vi "Set VeriStand Error.vi"(6 "message":string, 8 "error in (no error)":errorcluster, 9 "key":string, 10 "errCode":i32(ring)=-307828 items=["Success"=0, "NoProjectOpen"=-307992, "SequenceCompileError"=-307988, "SessionAlreadyDeployed"=-307984, "SessionNotDeployed"=-307982, "SequenceNotFoundInSession"=-307981, "StimulusProfileSessionLocked"=-307980, "EmptyNodeName"=-307930, "NodeAlreadyExistsByName"=-307926, "NumberOfCoefficientsOutOfRange"=-307884, "DownloadFileError"=-307872, "IncorrectLogFileName"=-307871, "LogTriggerConditionSyntaxError"=-307868, "DuplicateLogSessionName"=-307867, "LogSessionNotFound"=-307865, "ChannelLengthMismatch"=-307830, "NodeNotFoundDuringCompile"=-307829, "ChannelNodeRemoved"=-307828, "NotAChannel"=-307825, "NotAWaveform"=-307824, "STIFileError"=-307784, "DependenciesCycle"=-307783, "ChannelNotFoundInLogFile"=-307782, "ChannelGroupNotFoundInLogFile"=-307781, "GatewayNotOnLocalhost"=-307780, "NotEnoughDynamicDataSharingSpace"=-307738, "TargetMissingDataSharingDevice"=-307737, "ChannelMappingsSizeMismatch"=-307728, "DuplicateChannelAliasMappings"=-307711, "NotAnInlineCustomDevice"=-307710, "IncompatibleModel"=-307703, "ModelDimensionMismatch"=-307702, "SLSCChassisLoadFailed"=-307691, "TargetDisabled"=-307689, "MismatchedLengths"=-307687, "TargetInvalid"=-307686, "ParameterNotFound"=-307685, "ServerPortAlreadyInUse"=-307684, "TargetDisconnected"=-307682, "ServiceConfigurationFile"=-307681, "ModelParameterFileParseError"=-307680, "NoActionRequired"=-307677, "InputParameterInvalid"=-307676, "HostRunningDifferentSystemDefinition"=-307671, "ChannelNotScalable"=-307668, "ChannelCannotBeFaulted"=-307666, "ChannelNotWritable"=-307665, "ChannelNotReadable"=-307664, "Timeout"=-307663, "NodeNotFound"=-307662, "SystemDefinitionDeploymentFailure"=-307661, "SystemDefinitionDeploymentTimeout"=-307660, "EmptyPassword"=-307659, "SystemDefinitionAlreadyActive"=-307658, "InvalidConfigurationPassword"=-307657, "NoSystemDefinitionLoaded"=-307656, "ComponentNotAvailable"=-307655, "NotDeployed"=-307654, "InvalidFile"=-307653, "FailedServerConnection"=-307652, "FunctionNotSupported"=-307651, "UnexpectedError"=-307650, "UnmappedAlias"=-307617, "InvalidStreamConditionForDataType"=-307554, "WaveformDataTypeMismatch"=-307553, "InvalidDaqPluginFile"=-307526, "FileVersionUnsupported"=-307525], 11 "Custom Device Item Ref in":T1 format="%.0x") -> (0 "error out":errorcluster, 1 "VeriStand Error out":errorcluster, 3 "Custom Device Item Ref out":T1 format="%.0x")   [LabVIEW 2017, in "Routing and Faulting Scripting.lvlib"]
uses:
  Routing and Faulting Scripting.lvlib
  <vilib>/NI Veristand/Custom Device API/Custom Device Item Ref.ctl
  NationalInstruments.VeriStand.SystemStorage
  <vilib>/NI Veristand/Custom Device API/Custom Device API.lvlib
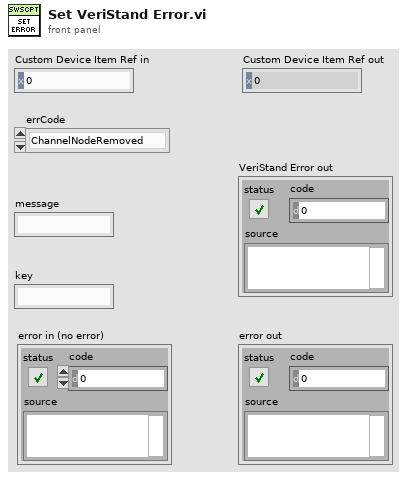
[diagram p1: front panel]
types:
  T1 = typedef "Custom Device API.lvlib/Custom Device Item Ref.ctl" = u64
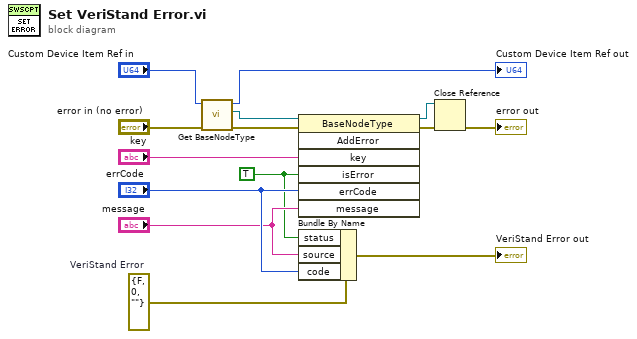
[diagram p0: block diagram]
diagram:
  w7 = errorcluster {"status"=FALSE, "code"=0, "source"=""}  # VeriStand Error
  w4 = TRUE ("isError")
  n1 = call "Get BaseNodeType.vi"("error in (no error)"="error in (no error)", "Item Ref in"="Custom Device Item Ref in") -> ("error out"=w14:errorcluster, "BaseNodeType"=w13:refnum<k24>, "Item Ref out"=→"Custom Device Item Ref out":T1)  [unwired: 7 in]
  n2 = invoke class="BaseNodeType" method="AddError"(reference=w13, error in=w14, "key"="key", "isError"=w4, "errCode"="errCode", "message"="message") -> (reference out=w11:refnum<k24>, error out=w12:errorcluster)  [unwired: 1 in, 5 out]
  n3 = Bundle By Name(cluster=w7, "status"=w4, "source"="message", "code"="errCode") -> (→"VeriStand Error out":errorcluster)
  n4 = Close Reference(reference=w11, error in (no error)=w12) -> (error out=→"error out":errorcluster)
